vi "Find value given key.vi"(10 "Key":string, 11 "request variables Input":cluster{"Key":string[], "Value":string[]}) -> (0 "Found":bool, 2 "Value":string)   [LabVIEW 2011, in "Design Server.lvlib"]
uses:
  AguaClara Design Server/Design Server.lvlib
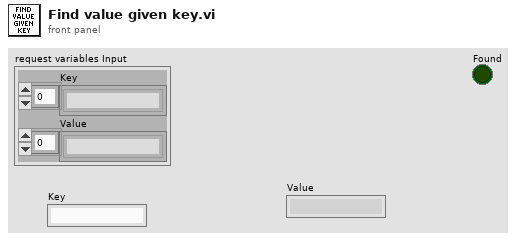
[diagram p1: front panel]
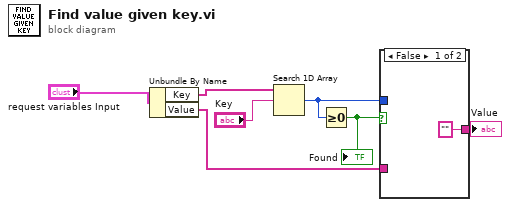
[diagram p0: block diagram]
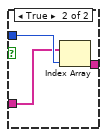
[diagram p2: hidden frame]
diagram:
  n1 = Unbundle By Name("request variables Input") -> ("Key"=w6:string[], "Value"=w4:string[])
  n2 = Search 1D Array(1D array=w6, element="Key") -> (index of element=w2:i32)  [unwired: 1 in]
  n3 = Greater Or Equal To 0?(x=w2) -> (x >= 0?=w1:bool)
  "Found" <- w1
  n4 = case shown="False" w1 {
    tunnel: w2 -> [_ w11]
    tunnel: w4 -> [_ w10]
    tunnel: ["" ("String") w9] -> w3
    frame False {
    }
    frame True {
      n5 = Index Array(array=w10, index=w11) -> (element=w9:string)
    }
  }
  "Value" <- w3
